vi "Read Functional Data (Multiple Correction).vi"(8 "error in (no error)":errorcluster, 10 "Channel No. (0)":i32, 11 "VISA resource name":refnum<visa-resource-name>) -> (0 "error out":errorcluster, 2 "Correction Data Array":dbl[](array[numeric]), 3 "VISA resource name out":refnum<visa-resource-name>)   [LabVIEW 2016, in "Agilent E4980.lvlib"]
doc: "Returns the open, short and load data for the multiple correction mode.\n\n<B>Notes:</B>\n(1) Returns 1206 data for the 201 test points, even if you turn off some frequency points. If there is no correction data, the instrument returns 0.0.\n\n(2) Elements of the array are: <open1 A>,<open1 B>,<short1 A>,<short1 B>, <load1 A>,<load1 B>,<open2 A>,<open2 B>,<short2 A>,<short2 B>, <load2 A>,<load2 B>,....,<open201 A>,<open201 B>,<short201 A>, <short201 B>,<load201 A>,<load201 B>"
uses:
  <instrlib>/Agilent E4980/Agilent E4980.lvlib
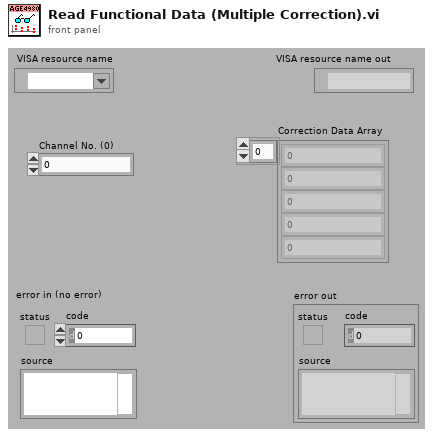
[diagram p1: front panel]
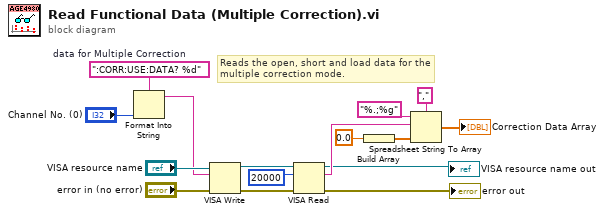
[diagram p0: block diagram]
diagram:
  w14 = ":CORR:USE:DATA? %d"  # data for Multiple Correction
  # "Reads the open, short and load data for the\nmultiple correction mode."
  n1 = Format Into String(format string=w14, "Channel No. (0)") -> (resulting string=w13:string)  [unwired: 2 in, 1 out]
  n2 = VISA Write(VISA resource name="VISA resource name", write buffer=w13, error in (no error)="error in (no error)") -> (VISA resource name out=w12:refnum<visa-resource-name>, error out=w11:errorcluster)  [unwired: 1 out]
  n3 = VISA Read(VISA resource name=w12, byte count=u32 20000, error in (no error)=w11) -> (VISA resource name out=→"VISA resource name out":refnum<visa-resource-name>, read buffer=w7:string, error out=→"error out":errorcluster)  [unwired: 1 out]
  n4 = Build Array(0.0) -> (w8:dbl[])
  n5 = Spreadsheet String To Array(delimiter (Tab)=",", format string="%.;%g", spreadsheet string=w7, array type (2D Dbl)=w8) -> (array=→"Correction Data Array":dbl[])
